vi "ChangeLanguage_old.vi"(10 "LanguageSelection":u16(ring) items=["Dansk", "English", "French"], 11 "VI Refnum":refnum<vi>) -> ()   [LabVIEW 2013, in "main.lvlib"]
uses:
  main.lvlib
  <vilib>/Utility/file.llb/Read From Spreadsheet File (string).vi
panel:
  out "Array 2":string[](array[string])
  out "appended array":string[][](array[string])
  out "Array":string[][](array[string])
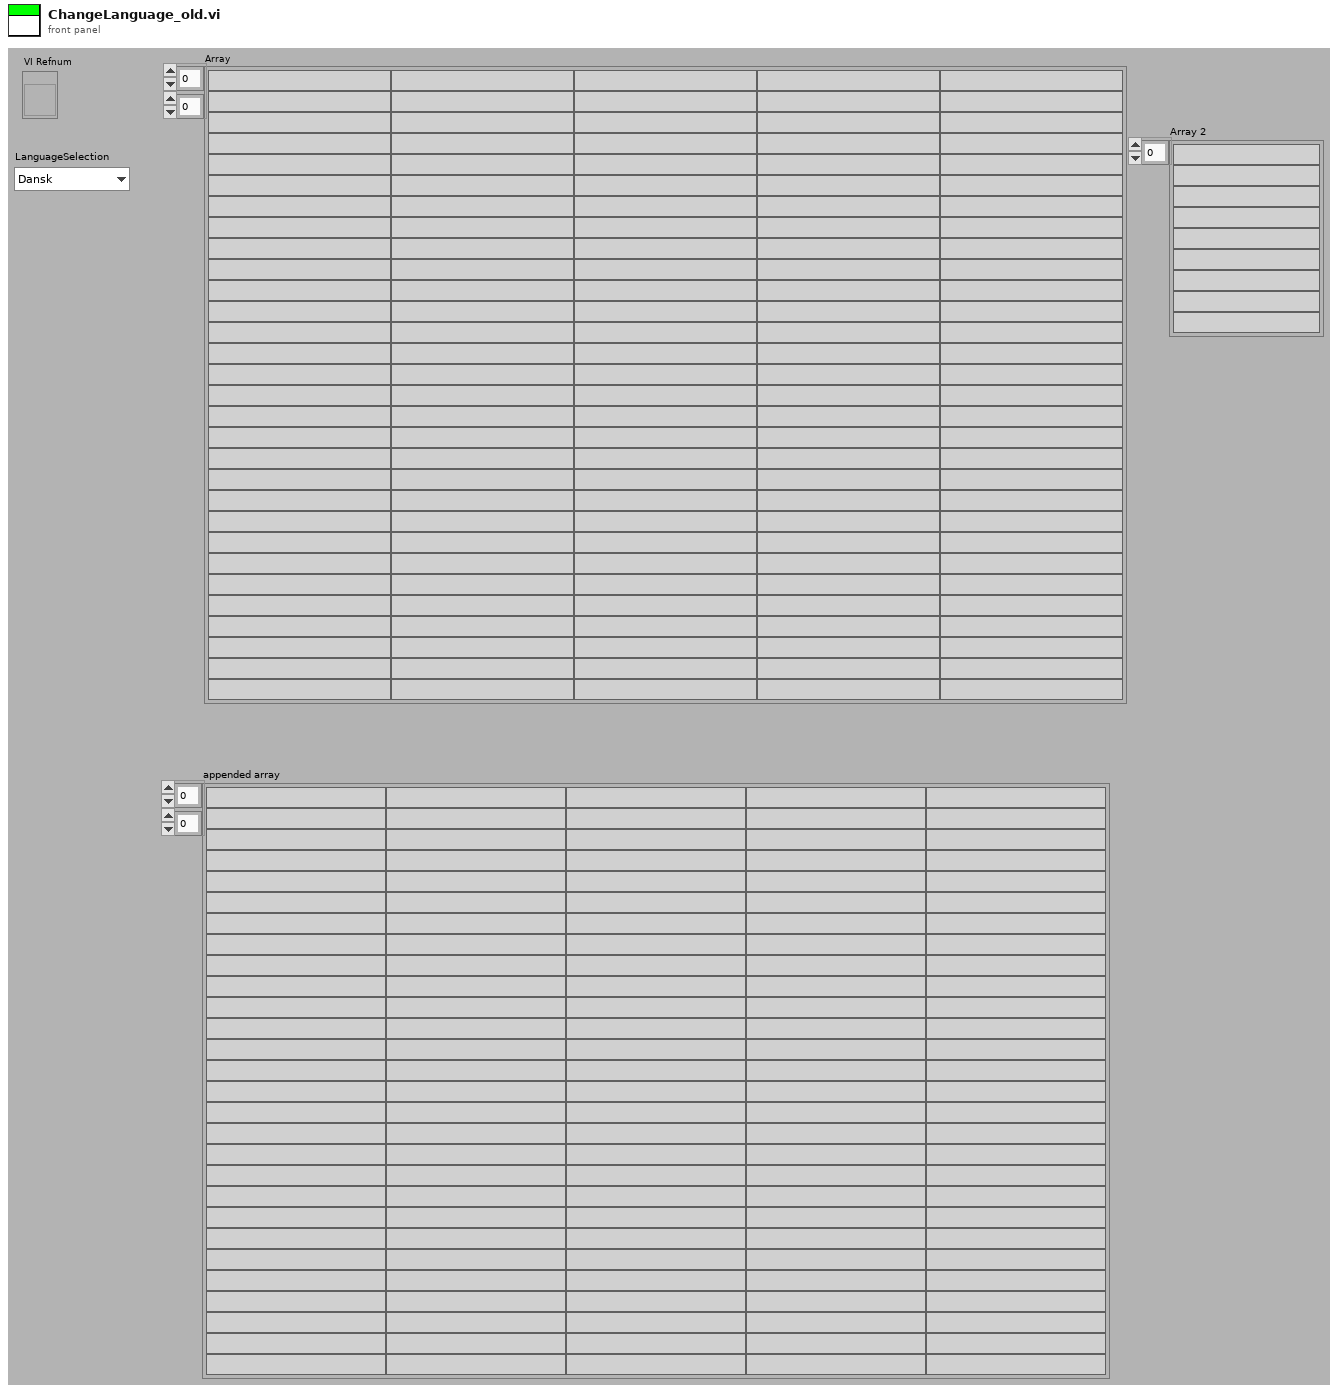
[diagram p1: front panel]
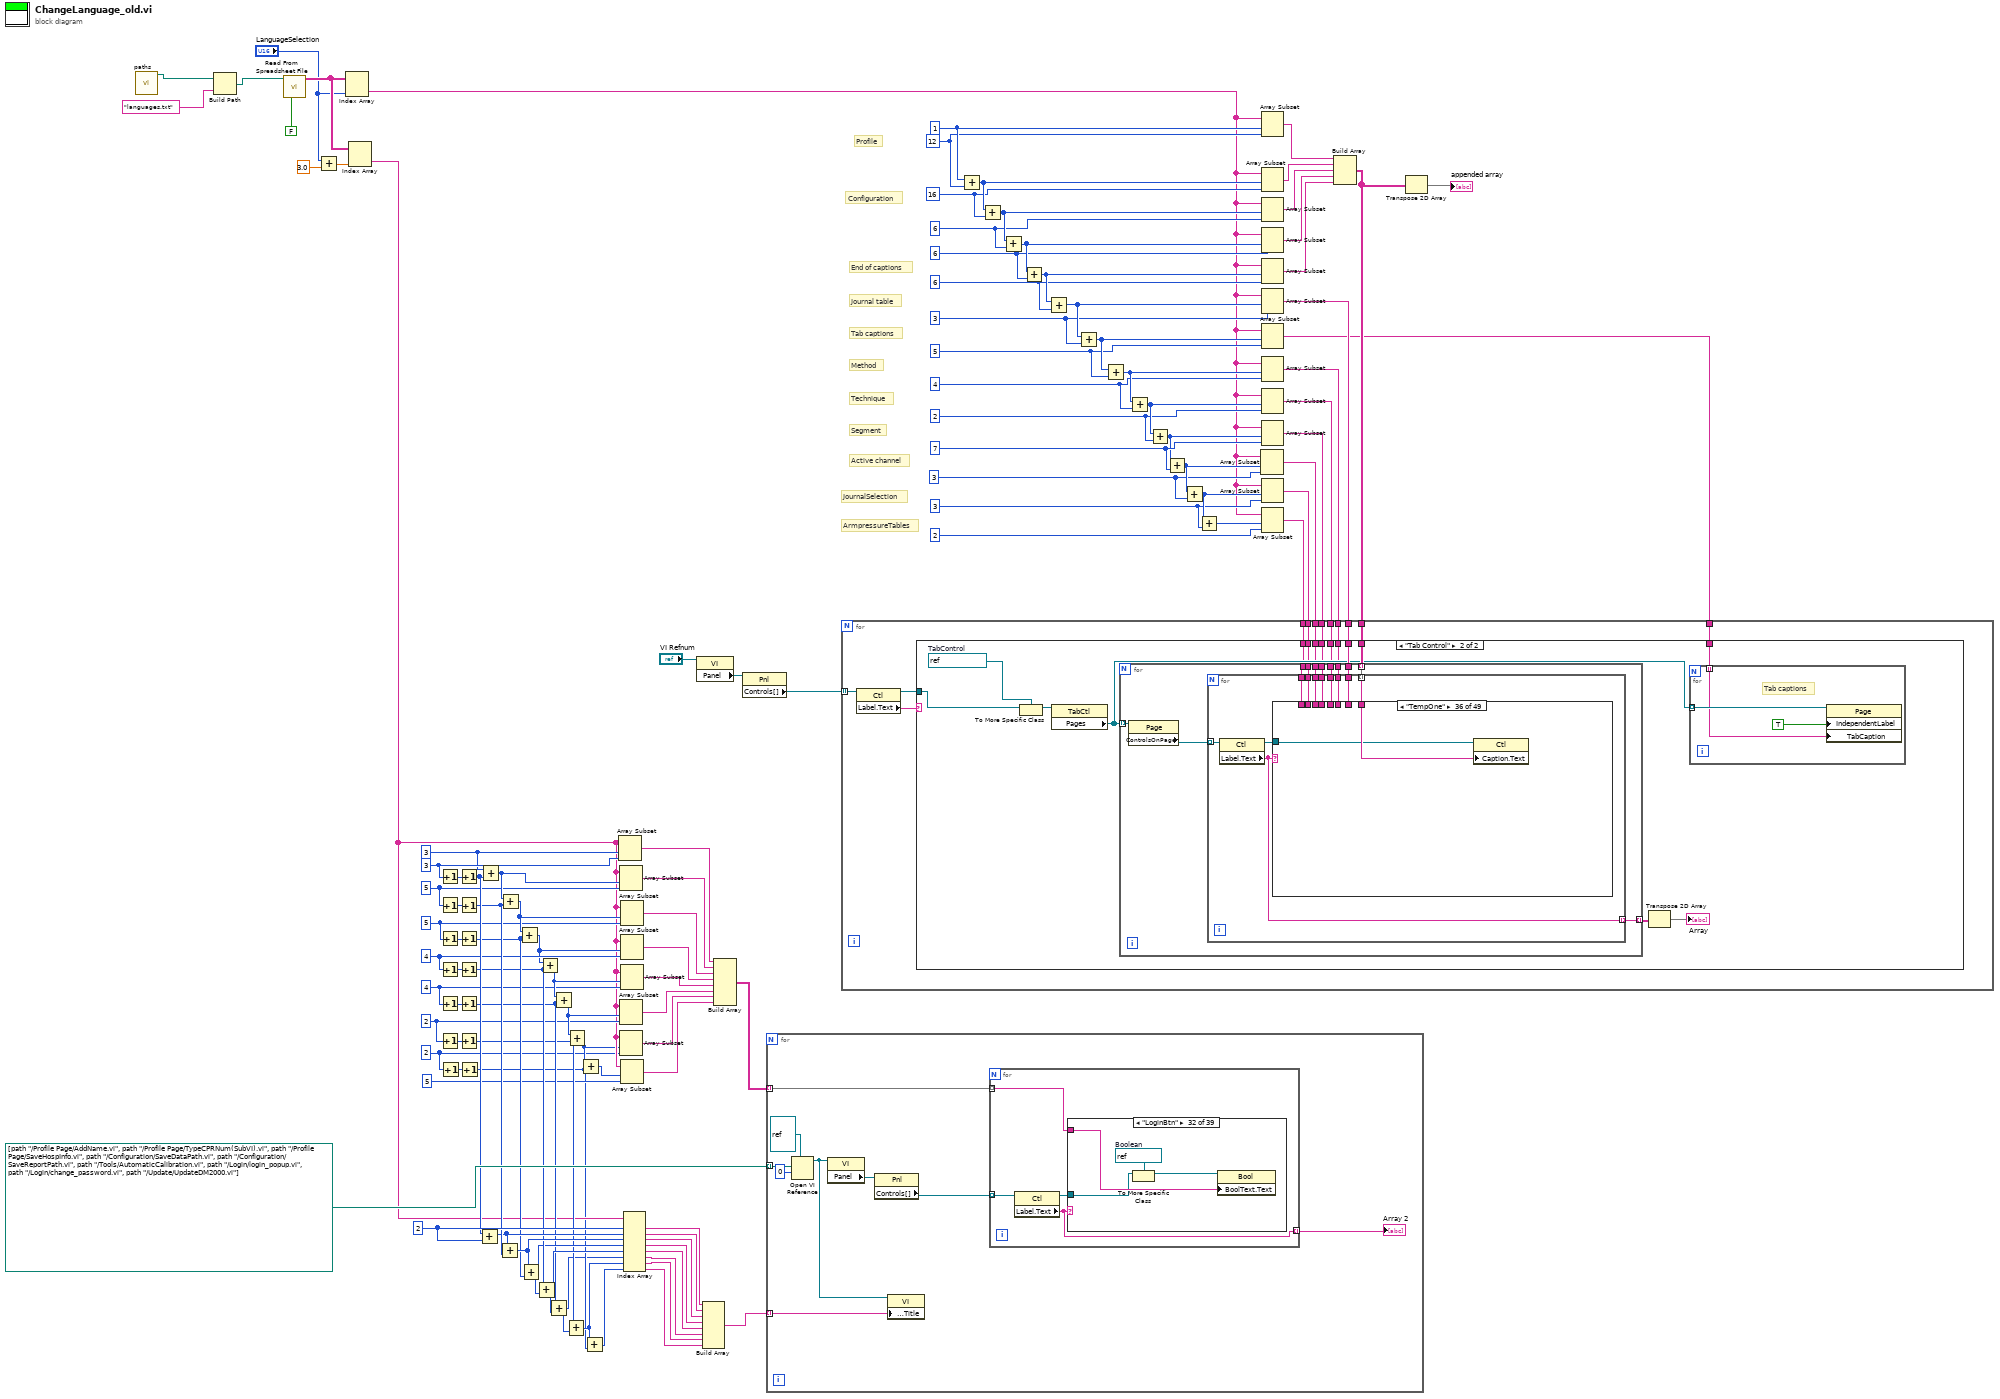
[diagram p0: block diagram]
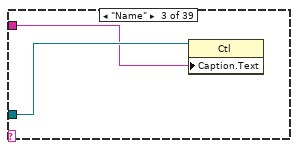
[diagram p4: hidden frame]
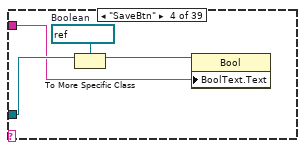
[diagram p5: hidden frame]
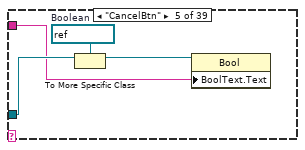
[diagram p6: hidden frame]
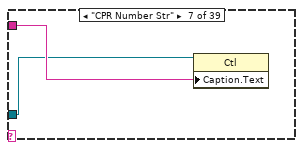
[diagram p8: hidden frame]
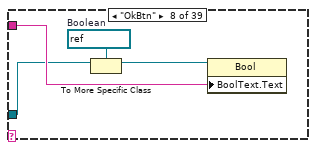
[diagram p9: hidden frame]
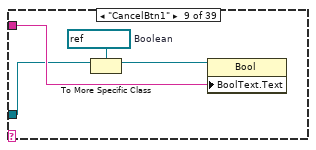
[diagram p10: hidden frame]
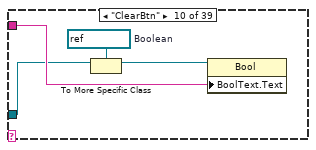
[diagram p11: hidden frame]
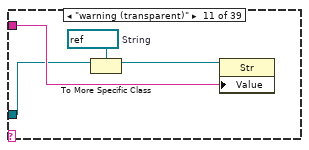
[diagram p12: hidden frame]
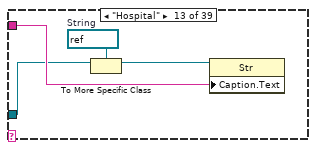
[diagram p14: hidden frame]
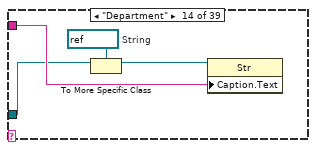
[diagram p15: hidden frame]
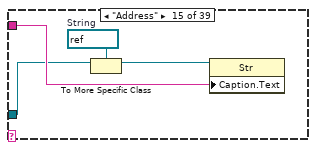
[diagram p16: hidden frame]
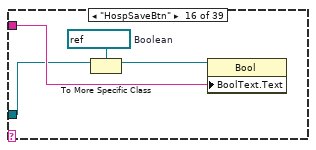
[diagram p17: hidden frame]
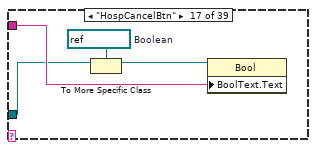
[diagram p18: hidden frame]
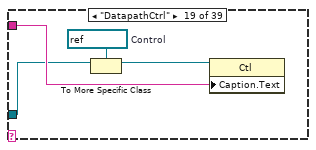
[diagram p20: hidden frame]
diagram:
  w3 = 3
  w17 = 2
  w8 = 3
  w31 = 7
  w33 = 2
  w36 = 4
  w25 = 2 ("length")
  w44 = 4 ("length")
  w53 = 4 ("length")
  w59 = 5 ("length")
  w66 = 5 ("length")
  w72 = 2 ("index")
  w71 = 3 ("length")
  w70 = 3 ("index")
  w39 = 5 ("length")
  w93 = 6 ("length")
  w95 = 16
  w87 = 3 ("length")
  w89 = 6 ("length")
  w91 = 6 ("length")
  w97 = 12 ("length")
  w98 = 1 ("index")
  # "Profile"
  # "Configuration"
  # "ArmpressureTables"
  # "JournalSelection"
  # "Tab captions"
  # "Active channel"
  # "Journal table"
  # "Segment"
  # "Technique"
  # "Method"
  # "End of captions"
  n1 = call "paths.vi"() -> ("PubAppData"=w28:path)  [unwired: 8 in, 3 out]
  n2 = Build Path(base path=w28, name or relative path="languages.txt") -> (appended path=w100:path)
  n3 = call-poly <vilib>:"Read From Spreadsheet File.vi"("transpose (no:F)"=FALSE, "file path (dialog if empty)"=w100) -> ("all rows"=w84:string[][])  [unwired: 5 in, 4 out]
  n4 = Add(x="LanguageSelection", y=3.0) -> (x+y=w83:dbl)
  n5 = Index Array(array=w84, index (col)="LanguageSelection") -> (element=w1:string[])  [unwired: 1 in]
  n6 = Index Array(array=w84, index (col)=w83) -> (element=w19:string[])  [unwired: 1 in]
  n7 = Increment(x=w71) -> (x+1=w73:i32)
  n8 = Increment(x=w66) -> (x+1=w68:i32)
  n9 = Increment(x=w59) -> (x+1=w61:i32)
  n10 = Increment(x=w53) -> (x+1=w54:i32)
  n11 = Increment(x=w44) -> (x+1=w46:i32)
  n12 = Increment(x=w25) -> (x+1=w26:i32)
  n13 = Increment(x=w17) -> (x+1=w22:i32)
  n14 = Increment(x=w73) -> (x+1=w69:i32)
  n15 = Increment(x=w68) -> (x+1=w64:i32)
  n16 = Increment(x=w61) -> (x+1=w57:i32)
  n17 = Increment(x=w54) -> (x+1=w51:i32)
  n18 = Increment(x=w46) -> (x+1=w43:i32)
  n19 = Increment(x=w26) -> (x+1=w23:i32)
  n20 = Increment(x=w22) -> (x+1=w15:i32)
  n21 = Add(x=w69, y=w72) -> (x+y=w63:i32)
  n22 = Add(x=w70, y=w69) -> (x+y=w67:i32)
  n23 = Add(x=w63, y=w64) -> (x+y=w58:i32)
  n24 = Add(x=w67, y=w64) -> (x+y=w60:i32)
  n25 = Add(x=w60, y=w57) -> (x+y=w52:i32)
  n26 = Add(x=w58, y=w57) -> (x+y=w50:i32)
  n27 = Add(x=w51, y=w50) -> (x+y=w47:i32)
  n28 = Add(x=w52, y=w51) -> (x+y=w45:i32)
  n29 = Add(x=w43, y=w47) -> (x+y=w14:i32)
  n30 = Add(x=w45, y=w43) -> (x+y=w27:i32)
  n31 = Add(x=w23, y=w14) -> (x+y=w16:i32)
  n32 = Add(x=w27, y=w23) -> (x+y=w18:i32)
  n33 = Add(x=w18, y=w15) -> (x+y=w20:i32)
  n34 = Add(x=w16, y=w15) -> (x+y=w13:i32)
  n35 = Array Subset(array=w19, index=w70, length=w71) -> (w80:string[])
  n36 = Array Subset(array=w19, index=w67, length=w66) -> (w79:string[])
  n37 = Array Subset(array=w19, index=w27, length=w25) -> (w41:string[])
  n38 = Array Subset(array=w19, index=w18, length=w17) -> (w24:string[])
  n39 = Array Subset(array=w19, index=w60, length=w59) -> (w65:string[])
  n40 = Array Subset(array=w19, index=w52, length=w53) -> (w55:string[])
  n41 = Array Subset(array=w19, index=w45, length=w44) -> (w48:string[])
  n42 = Array Subset(array=w19, index=w20, length=5) -> (w10:string[])
  n43 = Index Array(array=w19, index #1=w72, index #2=w63, index #3=w58, index #4=w50, index #5=w47, index #6=w14, index #7=w16, index #8=w13) -> (element #1=w76:string, element #2=w75:string, element #3=w62:string, element #4=w56:string, element #5=w49:string, element #6=w42:string, element #7=w12:string, element #8=w11:string)
  n44 = property class="VI"(reference="VI Refnum") -> ("Panel"=w111:refnum<vi>)  [unwired: 1 in, 2 out]
  n45 = Build Array(w76, w75, w62, w56, w49, w42, w12, w11) -> (w74:string[])
  n46 = Build Array(w80, w79, w65, w55, w48, w41, w24, w10) -> (w77:string[][])
  n47 = property class="Pnl"(reference=w111) -> ("Controls[]"=w110:refnum<vi>[])  [unwired: 1 in, 2 out]
  n48 = for {
    tunnel: path[] [path "../Profile Page/AddName.vi", path "../Profile Page/TypeCPRNum(SubVI).vi", path "../Profile Page/SaveHospInfo.vi", path "../Configuration/SaveDataPath.vi", path "../Configuration/SaveReportPath.vi", path "../Tools/AutomaticCalibration.vi", path "../Login/login_popup.vi", path "../Login/change_password.vi", path "../Update/UpdateDM2000.vi"] -> [w120] mode=indexing
    tunnel: w77 -> [w113] mode=indexing
    tunnel: w74 -> [w112] mode=indexing
    n49 = Open VI Reference(type specifier VI Refnum (for type only)=refnum<vi> refnum, vi path=w120, options=0) -> (vi reference=w114:refnum<vi>)  [unwired: 3 in, 1 out]
    n50 = property class="VI"(reference=w114) -> ("Panel"=w117:refnum<vi>)  [unwired: 1 in, 2 out]
    n51 = property class="Pnl"(reference=w117) -> ("Controls[]"=w119:refnum<vi>[])  [unwired: 1 in, 2 out]
    n52 = property class="VI"(reference=w114, "Front Panel.Title"=w112) -> ()  [unwired: 1 in, 2 out]
    n53 = for {
      tunnel: w119 -> [w124] mode=indexing
      tunnel: [w122] -> w118 mode=indexing
      tunnel: w113 -> [w121] mode=indexing
      n54 = property class="Ctl"(reference=w124) -> (reference out=w123:refnum<vi>, "Label.Text"=w122:string)  [unwired: 1 in, 1 out]
      n55 = case shown="\"LoginBtn\"" w122 {
        tunnel: w123 -> [_ _ w126 w129 w133 _ w135 w137 w141 w145 w149 _ w153 w157 w161 w165 w169 _ w173 w177 w181 w185 _ w189 w193 w197 w201 _ w205 w209 _ w213 w217 _ w221 w225 w229 w233 w237]
        tunnel: w121 -> [_ _ w125 w127 w131 _ w136 w138 w142 w146 w150 _ w154 w158 w162 w166 w170 _ w174 w178 w182 w186 _ w190 w194 w198 w202 _ w206 w210 _ w214 w218 _ w222 w226 w230 w234 w238]
        frame Default {
        }
        frame "/**AddName.vi" {
        }
        frame "Name" {
          n56 = property class="Ctl"(reference=w126, "Caption.Text"=w125) -> ()  [unwired: 1 in, 2 out]
        }
        frame "SaveBtn" {
          w130 = refnum<vi> refnum  # Boolean
          n57 = To More Specific Class(target class=w130, reference=w129) -> (specific class reference=w128:refnum<vi>)  [unwired: 1 in, 1 out]
          n58 = property class="Bool"(reference=w128, "BoolText.Text"=w127) -> ()  [unwired: 1 in, 2 out]
        }
        frame "CancelBtn" {
          w134 = refnum<vi> refnum  # Boolean
          n59 = To More Specific Class(target class=w134, reference=w133) -> (specific class reference=w132:refnum<vi>)  [unwired: 1 in, 1 out]
          n60 = property class="Bool"(reference=w132, "BoolText.Text"=w131) -> ()  [unwired: 1 in, 2 out]
        }
        frame "/**TypeCPRNum" {
        }
        frame "CPR Number Str" {
          n61 = property class="Ctl"(reference=w135, "Caption.Text"=w136) -> ()  [unwired: 1 in, 2 out]
        }
        frame "OkBtn" {
          w140 = refnum<vi> refnum  # Boolean
          n62 = To More Specific Class(target class=w140, reference=w137) -> (specific class reference=w139:refnum<vi>)  [unwired: 1 in, 1 out]
          n63 = property class="Bool"(reference=w139, "BoolText.Text"=w138) -> ()  [unwired: 1 in, 2 out]
        }
        frame "CancelBtn1" {
          w144 = refnum<vi> refnum  # Boolean
          n64 = To More Specific Class(target class=w144, reference=w141) -> (specific class reference=w143:refnum<vi>)  [unwired: 1 in, 1 out]
          n65 = property class="Bool"(reference=w143, "BoolText.Text"=w142) -> ()  [unwired: 1 in, 2 out]
        }
        frame "ClearBtn" {
          w148 = refnum<vi> refnum  # Boolean
          n66 = To More Specific Class(target class=w148, reference=w145) -> (specific class reference=w147:refnum<vi>)  [unwired: 1 in, 1 out]
          n67 = property class="Bool"(reference=w147, "BoolText.Text"=w146) -> ()  [unwired: 1 in, 2 out]
        }
        frame "warning (transparent)" {
          w152 = refnum<vi> refnum  # String
          n68 = To More Specific Class(target class=w152, reference=w149) -> (specific class reference=w151:refnum<vi>)  [unwired: 1 in, 1 out]
          n69 = property class="Str"(reference=w151, "Value"=w150) -> ()  [unwired: 1 in, 2 out]
        }
        frame "/***HospInfo" {
        }
        frame "Hospital" {
          w156 = refnum<vi> refnum  # String
          n70 = To More Specific Class(target class=w156, reference=w153) -> (specific class reference=w155:refnum<vi>)  [unwired: 1 in, 1 out]
          n71 = property class="Str"(reference=w155, "Caption.Text"=w154) -> ()  [unwired: 1 in, 2 out]
        }
        frame "Department" {
          w160 = refnum<vi> refnum  # String
          n72 = To More Specific Class(target class=w160, reference=w157) -> (specific class reference=w159:refnum<vi>)  [unwired: 1 in, 1 out]
          n73 = property class="Str"(reference=w159, "Caption.Text"=w158) -> ()  [unwired: 1 in, 2 out]
        }
        frame "Address" {
          w164 = refnum<vi> refnum  # String
          n74 = To More Specific Class(target class=w164, reference=w161) -> (specific class reference=w163:refnum<vi>)  [unwired: 1 in, 1 out]
          n75 = property class="Str"(reference=w163, "Caption.Text"=w162) -> ()  [unwired: 1 in, 2 out]
        }
        frame "HospSaveBtn" {
          w168 = refnum<vi> refnum  # Boolean
          n76 = To More Specific Class(target class=w168, reference=w165) -> (specific class reference=w167:refnum<vi>)  [unwired: 1 in, 1 out]
          n77 = property class="Bool"(reference=w167, "BoolText.Text"=w166) -> ()  [unwired: 1 in, 2 out]
        }
        frame "HospCancelBtn" {
          w172 = refnum<vi> refnum  # Boolean
          n78 = To More Specific Class(target class=w172, reference=w169) -> (specific class reference=w171:refnum<vi>)  [unwired: 1 in, 1 out]
          n79 = property class="Bool"(reference=w171, "BoolText.Text"=w170) -> ()  [unwired: 1 in, 2 out]
        }
        frame "/***SaveDataPath" {
        }
        frame "DatapathCtrl" {
          w176 = refnum<vi> refnum  # Control
          n80 = To More Specific Class(target class=w176, reference=w173) -> (specific class reference=w175:refnum<vi>)  [unwired: 1 in, 1 out]
          n81 = property class="Ctl"(reference=w175, "Caption.Text"=w174) -> ()  [unwired: 1 in, 2 out]
        }
        frame "DatapathSaveBtn" {
          w180 = refnum<vi> refnum  # Boolean
          n82 = To More Specific Class(target class=w180, reference=w177) -> (specific class reference=w179:refnum<vi>)  [unwired: 1 in, 1 out]
          n83 = property class="Bool"(reference=w179, "BoolText.Text"=w178) -> ()  [unwired: 1 in, 2 out]
        }
        frame "DatapathCancelBtn" {
          w184 = refnum<vi> refnum  # Boolean
          n84 = To More Specific Class(target class=w184, reference=w181) -> (specific class reference=w183:refnum<vi>)  [unwired: 1 in, 1 out]
          n85 = property class="Bool"(reference=w183, "BoolText.Text"=w182) -> ()  [unwired: 1 in, 2 out]
        }
        frame "String (transparent)" {
          w188 = refnum<vi> refnum  # String
          n86 = To More Specific Class(target class=w188, reference=w185) -> (specific class reference=w187:refnum<vi>)  [unwired: 1 in, 1 out]
          n87 = property class="Str"(reference=w187, "Caption.Text"=w186) -> ()  [unwired: 1 in, 2 out]
        }
        frame "/***SaveReportPath" {
        }
        frame "ReportPathCtrl" {
          w192 = refnum<vi> refnum  # Control
          n88 = To More Specific Class(target class=w192, reference=w189) -> (specific class reference=w191:refnum<vi>)  [unwired: 1 in, 1 out]
          n89 = property class="Ctl"(reference=w191, "Caption.Text"=w190) -> ()  [unwired: 1 in, 2 out]
        }
        frame "ReportSaveBtn" {
          w196 = refnum<vi> refnum  # Boolean
          n90 = To More Specific Class(target class=w196, reference=w193) -> (specific class reference=w195:refnum<vi>)  [unwired: 1 in, 1 out]
          n91 = property class="Bool"(reference=w195, "BoolText.Text"=w194) -> ()  [unwired: 1 in, 2 out]
        }
        frame "ReportCancelBtn" {
          w200 = refnum<vi> refnum  # Boolean
          n92 = To More Specific Class(target class=w200, reference=w197) -> (specific class reference=w199:refnum<vi>)  [unwired: 1 in, 1 out]
          n93 = property class="Bool"(reference=w199, "BoolText.Text"=w198) -> ()  [unwired: 1 in, 2 out]
        }
        frame "ReportString (transparent)" {
          w204 = refnum<vi> refnum  # String
          n94 = To More Specific Class(target class=w204, reference=w201) -> (specific class reference=w203:refnum<vi>)  [unwired: 1 in, 1 out]
          n95 = property class="Str"(reference=w203, "Caption.Text"=w202) -> ()  [unwired: 1 in, 2 out]
        }
        frame "/***AutomaticCalibration" {
        }
        frame "CalibrationStopBtn" {
          w208 = refnum<vi> refnum  # Boolean
          n96 = To More Specific Class(target class=w208, reference=w205) -> (specific class reference=w207:refnum<vi>)  [unwired: 1 in, 1 out]
          n97 = property class="Bool"(reference=w207, "BoolText.Text"=w206) -> ()  [unwired: 1 in, 2 out]
        }
        frame "CalibrationCancelBtn" {
          w212 = refnum<vi> refnum  # Boolean
          n98 = To More Specific Class(target class=w212, reference=w209) -> (specific class reference=w211:refnum<vi>)  [unwired: 1 in, 1 out]
          n99 = property class="Bool"(reference=w211, "BoolText.Text"=w210) -> ()  [unwired: 1 in, 2 out]
        }
        frame "/**Login**/" {
        }
        frame "LoginBtn" {
          w216 = refnum<vi> refnum  # Boolean
          n100 = To More Specific Class(target class=w216, reference=w213) -> (specific class reference=w215:refnum<vi>)  [unwired: 1 in, 1 out]
          n101 = property class="Bool"(reference=w215, "BoolText.Text"=w214) -> ()  [unwired: 1 in, 2 out]
        }
        frame "LoginCancelBtn" {
          w220 = refnum<vi> refnum  # Boolean
          n102 = To More Specific Class(target class=w220, reference=w217) -> (specific class reference=w219:refnum<vi>)  [unwired: 1 in, 1 out]
          n103 = property class="Bool"(reference=w219, "BoolText.Text"=w218) -> ()  [unwired: 1 in, 2 out]
        }
        frame "/**ChangePassword**/" {
        }
        frame "PresentPassword" {
          w224 = refnum<vi> refnum  # String
          n104 = To More Specific Class(target class=w224, reference=w221) -> (specific class reference=w223:refnum<vi>)  [unwired: 1 in, 1 out]
          n105 = property class="Str"(reference=w223, "Caption.Text"=w222) -> ()  [unwired: 1 in, 2 out]
        }
        frame "NewPassword" {
          w228 = refnum<vi> refnum  # String
          n106 = To More Specific Class(target class=w228, reference=w225) -> (specific class reference=w227:refnum<vi>)  [unwired: 1 in, 1 out]
          n107 = property class="Str"(reference=w227, "Caption.Text"=w226) -> ()  [unwired: 1 in, 2 out]
        }
        frame "RetypePassword" {
          w232 = refnum<vi> refnum  # String
          n108 = To More Specific Class(target class=w232, reference=w229) -> (specific class reference=w231:refnum<vi>)  [unwired: 1 in, 1 out]
          n109 = property class="Str"(reference=w231, "Caption.Text"=w230) -> ()  [unwired: 1 in, 2 out]
        }
        frame "Submit" {
          w236 = refnum<vi> refnum  # Boolean
          n110 = To More Specific Class(target class=w236, reference=w233) -> (specific class reference=w235:refnum<vi>)  [unwired: 1 in, 1 out]
          n111 = property class="Bool"(reference=w235, "BoolText.Text"=w234) -> ()  [unwired: 1 in, 2 out]
        }
        frame "Cancel" {
          w240 = refnum<vi> refnum  # Boolean
          n112 = To More Specific Class(target class=w240, reference=w237) -> (specific class reference=w239:refnum<vi>)  [unwired: 1 in, 1 out]
          n113 = property class="Bool"(reference=w239, "BoolText.Text"=w238) -> ()  [unwired: 1 in, 2 out]
        }
      }
    }
    "Array 2" <- w118
  }
  n114 = Add(x=w98, y=w97) -> (x+y=w96:i32)
  n115 = Add(x=w96, y=w95) -> (x+y=w94:i32)
  n116 = Add(x=w94, y=w93) -> (x+y=w92:i32)
  n117 = Add(x=w92, y=w91) -> (x+y=w90:i32)
  n118 = Add(x=w90, y=w89) -> (x+y=w88:i32)
  n119 = Add(x=w88, y=w87) -> (x+y=w40:i32)
  n120 = Add(x=w40, y=w39) -> (x+y=w37:i32)
  n121 = Add(x=w37, y=w36) -> (x+y=w34:i32)
  n122 = Add(x=w34, y=w33) -> (x+y=w30:i32)
  n123 = Add(x=w30, y=w31) -> (x+y=w9:i32)
  n124 = Add(x=w9, y=w8) -> (x+y=w4:i32)
  n125 = Add(x=w4, y=w3) -> (x+y=w6:i32)
  n126 = Array Subset(array=w1, index=w9, length=w8) -> (w29:string[])
  n127 = Array Subset(array=w1, index=w98, length=w97) -> (w108:string[])
  n128 = Array Subset(array=w1, index=w96, length=w95) -> (w107:string[])
  n129 = Array Subset(array=w1, index=w94, length=w93) -> (w106:string[])
  n130 = Array Subset(array=w1, index=w92, length=w91) -> (w105:string[])
  n131 = Array Subset(array=w1, index=w90, length=w89) -> (w104:string[])
  n132 = Array Subset(array=w1, index=w88, length=w87) -> (w101:string[])
  n133 = Array Subset(array=w1, index=w40, length=w39) -> (w86:string[])
  n134 = Array Subset(array=w1, index=w37, length=w36) -> (w38:string[])
  n135 = Array Subset(array=w1, index=w34, length=w33) -> (w35:string[])
  n136 = Array Subset(array=w1, index=w30, length=w31) -> (w32:string[])
  n137 = Array Subset(array=w1, index=w4, length=w3) -> (w7:string[])
  n138 = Array Subset(array=w1, index=w6, length=2) -> (w2:string[])
  n139 = Build Array(w108, w107, w106, w105, w104) -> (w102:string[][])
  n140 = for {
    tunnel: w110 -> [w252] mode=indexing
    tunnel: w102 -> [w249]
    tunnel: w101 -> [w248]
    tunnel: w86 -> [w247]
    tunnel: w38 -> [w246]
    tunnel: w35 -> [w245]
    tunnel: w32 -> [w244]
    tunnel: w29 -> [w243]
    tunnel: w7 -> [w242]
    tunnel: w2 -> [w241]
    n141 = property class="Ctl"(reference=w252) -> (reference out=w251:refnum<vi>, "Label.Text"=w250:string)  [unwired: 1 in, 1 out]
    n142 = case shown="\"Tab Control\"" w250 {
      tunnel: w251 -> [_ w267]
      tunnel: w249 -> [_ w262]
      tunnel: w248 -> [_ w261]
      tunnel: w247 -> [_ w259]
      tunnel: w246 -> [_ w258]
      tunnel: w245 -> [_ w257]
      tunnel: w244 -> [_ w256]
      tunnel: w243 -> [_ w255]
      tunnel: w242 -> [_ w254]
      tunnel: w241 -> [_ w253]
      frame "False", Default {
      }
      frame "Tab Control" {
        w266 = refnum<vi> refnum  # TabControl
        n143 = To More Specific Class(target class=w266, reference=w267) -> (specific class reference=w265:refnum<vi>)  [unwired: 1 in, 1 out]
        n144 = property class="TabCtl"(reference=w265) -> ("Pages"=w260:refnum<vi>[])  [unwired: 1 in, 2 out]
        n145 = for {
          tunnel: w260 -> [w277] mode=indexing
          tunnel: [w280] -> w264 mode=indexing
          tunnel: w262 -> [w279] mode=indexing
          tunnel: w261 -> [w278]
          tunnel: w258 -> [w276]
          tunnel: w257 -> [w275]
          tunnel: w256 -> [w274]
          tunnel: w255 -> [w273]
          tunnel: w254 -> [w272]
          tunnel: w253 -> [w271]
          n146 = property class="Page"(reference=w277) -> ("ControlsOnPage"=w281:refnum<vi>[])  [unwired: 1 in, 2 out]
          n147 = for {
            tunnel: w281 -> [w292] mode=indexing
            tunnel: [w291] -> w280 mode=indexing
            tunnel: w279 -> [w289] mode=indexing
            tunnel: w278 -> [w288]
            tunnel: w276 -> [w287]
            tunnel: w275 -> [w286]
            tunnel: w274 -> [w285]
            tunnel: w273 -> [w284]
            tunnel: w272 -> [w283]
            tunnel: w271 -> [w282]
            n148 = property class="Ctl"(reference=w292) -> (reference out=w290:refnum<vi>, "Label.Text"=w291:string)  [unwired: 1 in, 1 out]
            n149 = case shown="\"TempOne\"" w291 {
              tunnel: w290 -> [_ w295 w298 w302 w303 w309 w312 w316 w318 w322 w324 w326 w328 w331 w336 w341 w345 w347 w351 w356 w359 w361 w363 w365 w369 w373 w377 w380 w382 w384 w386 w388 w390 w392 w394 w396 w398 w400 w402 w404 w408 w413 w415 w419 w424 w427 w431 w435 w439]
              tunnel: w289 -> [_ w296 w300 w301 w306 w308 w311 w315 w320 w321 w323 w325 w327 w330 w335 w340 w344 w346 w349 w354 w358 w360 w362 w364 w368 w372 w376 w381 w383 w385 w387 w389 w391 w393 w395 w397 w399 w401 w403 w405 w410 w412 w416 w420 w425 w426 w430 _ w440]
              tunnel: w288 -> [_ _ _ _ _ _ _ _ _ _ _ _ _ _ _ _ _ _ _ _ _ _ _ _ _ _ _ _ _ _ _ _ _ _ _ _ _ _ _ _ _ _ _ _ _ _ _ w434 _]
              tunnel: w287 -> [_ _ _ _ _ _ _ _ _ _ _ _ _ w329 _ _ _ _ _ _ _ _ _ _ _ _ _ _ _ _ _ _ _ _ _ _ _ _ _ _ _ _ _ _ _ _ _ _ _]
              tunnel: w286 -> [_ _ _ _ _ _ _ _ _ _ _ _ _ _ w334 _ _ _ _ _ _ _ _ _ _ _ _ _ _ _ _ _ _ _ _ _ _ _ _ _ _ _ _ _ _ _ _ _ _]
              tunnel: w285 -> [_ _ _ _ _ _ _ _ _ _ _ _ _ _ _ w339 _ _ _ _ _ _ _ _ _ _ _ _ _ _ _ _ _ _ _ _ _ _ _ _ _ _ _ _ _ _ _ _ _]
              tunnel: w284 -> [_ _ _ _ _ _ _ _ _ _ _ _ _ _ _ _ _ _ _ _ _ _ _ _ _ _ _ _ _ _ _ _ _ _ _ _ _ _ _ _ w406 _ _ _ _ _ _ _ _]
              tunnel: w283 -> [_ _ _ _ _ _ _ _ _ _ _ _ _ _ _ _ _ _ _ _ _ _ _ _ _ _ _ _ _ _ _ _ _ _ _ _ _ _ _ _ _ _ _ _ w421 _ _ _ _]
              tunnel: w282 -> [_ _ _ _ _ _ _ _ _ _ _ _ _ _ _ _ _ _ w348 w353 _ _ _ _ _ _ _ _ _ _ _ _ _ _ _ _ _ _ _ _ _ _ _ _ _ _ _ _ _]
              frame Default {
              }
              frame "ListboxCpr" {
                w294 = refnum<vi> refnum  # ListBox
                n150 = To More Specific Class(target class=w294, reference=w295) -> (specific class reference=w293:refnum<vi>)  [unwired: 1 in, 1 out]
                n151 = property class="LstBox"(reference=w293, "ColHdr"=w296) -> ()  [unwired: 1 in, 2 out]
              }
              frame "SelectCprBtn" {
                w299 = refnum<vi> refnum  # Boolean
                n152 = To More Specific Class(target class=w299, reference=w298) -> (specific class reference=w297:refnum<vi>)  [unwired: 1 in, 1 out]
                n153 = property class="Bool"(reference=w297, "BoolText.Text"=w300) -> ()  [unwired: 1 in, 2 out]
              }
              frame "Name" {
                n154 = property class="Ctl"(reference=w302, "Caption.Text"=w301) -> ()  [unwired: 1 in, 2 out]
              }
              frame "AddCprBtn" {
                w305 = refnum<vi> refnum  # Boolean
                n155 = To More Specific Class(target class=w305, reference=w303) -> (specific class reference=w304:refnum<vi>)  [unwired: 1 in, 1 out]
                n156 = property class="Bool"(reference=w304, "BoolText.Text"=w306) -> ()  [unwired: 1 in, 2 out]
              }
              frame "ListboxOperator" {
                w310 = refnum<vi> refnum  # ListBox
                n157 = To More Specific Class(target class=w310, reference=w309) -> (specific class reference=w307:refnum<vi>)  [unwired: 1 in, 1 out]
                n158 = property class="LstBox"(reference=w307, "ColHdr"=w308) -> ()  [unwired: 1 in, 2 out]
              }
              frame "ListboxDoctor" {
                w314 = refnum<vi> refnum  # ListBox
                n159 = To More Specific Class(target class=w314, reference=w312) -> (specific class reference=w313:refnum<vi>)  [unwired: 1 in, 1 out]
                n160 = property class="LstBox"(reference=w313, "ColHdr"=w311) -> ()  [unwired: 1 in, 2 out]
              }
              frame "HospitalName" {
                n161 = property class="Ctl"(reference=w316, "Caption.Text"=w315) -> ()  [unwired: 1 in, 2 out]
              }
              frame "EditHospInfo" {
                w319 = refnum<vi> refnum  # Boolean
                n162 = To More Specific Class(target class=w319, reference=w318) -> (specific class reference=w317:refnum<vi>)  [unwired: 1 in, 1 out]
                n163 = property class="Bool"(reference=w317, "BoolText.Text"=w320) -> ()  [unwired: 1 in, 2 out]
              }
              frame "HospitalAddress" {
                n164 = property class="Ctl"(reference=w322, "Caption.Text"=w321) -> ()  [unwired: 1 in, 2 out]
              }
              frame "CommentString" {
                n165 = property class="Ctl"(reference=w324, "Caption.Text"=w323) -> ()  [unwired: 1 in, 2 out]
              }
              frame "HospitalDepartment" {
                n166 = property class="Ctl"(reference=w326, "Caption.Text"=w325) -> ()  [unwired: 1 in, 2 out]
              }
              frame "SearchCprField" {
                n167 = property class="Ctl"(reference=w328, "Caption.Text"=w327) -> ()  [unwired: 1 in, 2 out]
              }
              frame "ListboxMeasurementMeth" {
                w333 = refnum<vi> refnum  # ListBox
                n168 = To More Specific Class(target class=w333, reference=w331) -> (specific class reference=w332:refnum<vi>)  [unwired: 1 in, 1 out]
                n169 = property class="LstBox"(reference=w332, "Caption.Text"=w330, "Item Names"=w329) -> ()  [unwired: 1 in, 2 out]
              }
              frame "ListboxMeasurementTechnique" {
                w338 = refnum<vi> refnum  # ListBox
                n170 = To More Specific Class(target class=w338, reference=w336) -> (specific class reference=w337:refnum<vi>)  [unwired: 1 in, 1 out]
                n171 = property class="LstBox"(reference=w337, "Caption.Text"=w335, "Item Names"=w334) -> ()  [unwired: 1 in, 2 out]
              }
              frame "ListboxMeasurementArea" {
                w343 = refnum<vi> refnum  # ListBox
                n172 = To More Specific Class(target class=w343, reference=w341) -> (specific class reference=w342:refnum<vi>)  [unwired: 1 in, 1 out]
                n173 = property class="LstBox"(reference=w342, "Caption.Text"=w340, "Item Names"=w339) -> ()  [unwired: 1 in, 2 out]
              }
              frame "ListboxRightSegmentNr" {
                n174 = property class="Ctl"(reference=w345, "Caption.Text"=w344) -> ()  [unwired: 1 in, 2 out]
              }
              frame "ListboxLeftSegmentNr" {
                n175 = property class="Ctl"(reference=w347, "Caption.Text"=w346) -> ()  [unwired: 1 in, 2 out]
              }
              frame "RightArmPressureTable" {
                w350 = refnum<vi> refnum  # Table
                n176 = To More Specific Class(target class=w350, reference=w351) -> (specific class reference=w352:refnum<vi>)  [unwired: 1 in, 1 out]
                n177 = property class="Tbl"(reference=w352, "Caption.Text"=w349, "Column Headers[]"=w348) -> ()  [unwired: 1 in, 2 out]
              }
              frame "LeftArmPressureTable" {
                w355 = refnum<vi> refnum  # Table
                n178 = To More Specific Class(target class=w355, reference=w356) -> (specific class reference=w357:refnum<vi>)  [unwired: 1 in, 1 out]
                n179 = property class="Tbl"(reference=w357, "Caption.Text"=w354, "Column Headers[]"=w353) -> ()  [unwired: 1 in, 2 out]
              }
              frame "Puls" {
                n180 = property class="Ctl"(reference=w359, "Caption.Text"=w358) -> ()  [unwired: 1 in, 2 out]
              }
              frame "HeightAdjustmentInt" {
                n181 = property class="Ctl"(reference=w361, "Caption.Text"=w360) -> ()  [unwired: 1 in, 2 out]
              }
              frame "Segment Number" {
                n182 = property class="Ctl"(reference=w363, "Caption.Text"=w362) -> ()  [unwired: 1 in, 2 out]
              }
              frame "SaveArmPressureBtn" {
                w367 = refnum<vi> refnum  # Boolean
                n183 = To More Specific Class(target class=w367, reference=w365) -> (specific class reference=w366:refnum<vi>)  [unwired: 1 in, 1 out]
                n184 = property class="Bool"(reference=w366, "BoolText.Text"=w364) -> ()  [unwired: 1 in, 2 out]
              }
              frame "EditDataPath" {
                w371 = refnum<vi> refnum  # Boolean
                n185 = To More Specific Class(target class=w371, reference=w369) -> (specific class reference=w370:refnum<vi>)  [unwired: 1 in, 1 out]
                n186 = property class="Bool"(reference=w370, "BoolText.Text"=w368) -> ()  [unwired: 1 in, 2 out]
              }
              frame "ReportPathBtn" {
                w375 = refnum<vi> refnum  # Boolean
                n187 = To More Specific Class(target class=w375, reference=w373) -> (specific class reference=w374:refnum<vi>)  [unwired: 1 in, 1 out]
                n188 = property class="Bool"(reference=w374, "BoolText.Text"=w372) -> ()  [unwired: 1 in, 2 out]
              }
              frame "ChangeLanguage" {
                w379 = refnum<vi> refnum  # Ring
                n189 = To More Specific Class(target class=w379, reference=w377) -> (specific class reference=w378:refnum<vi>)  [unwired: 1 in, 1 out]
                n190 = property class="Ring"(reference=w378, "Caption.Text"=w376) -> ()  [unwired: 1 in, 2 out]
              }
              frame "Arm1" {
                n191 = property class="Ctl"(reference=w380, "Value"=w381) -> ()  [unwired: 1 in, 2 out]
              }
              frame "Arm2" {
                n192 = property class="Ctl"(reference=w382, "Value"=w383) -> ()  [unwired: 1 in, 2 out]
              }
              frame "Right1" {
                n193 = property class="Ctl"(reference=w384, "Value"=w385) -> ()  [unwired: 1 in, 2 out]
              }
              frame "Left1" {
                n194 = property class="Ctl"(reference=w386, "Value"=w387) -> ()  [unwired: 1 in, 2 out]
              }
              frame "Right2" {
                n195 = property class="Ctl"(reference=w388, "Value"=w389) -> ()  [unwired: 1 in, 2 out]
              }
              frame "Left2" {
                n196 = property class="Ctl"(reference=w390, "Value"=w391) -> ()  [unwired: 1 in, 2 out]
              }
              frame "SettingsString" {
                n197 = property class="Ctl"(reference=w392, "Value"=w393) -> ()  [unwired: 1 in, 2 out]
              }
              frame "AdditionalInfoString" {
                n198 = property class="Ctl"(reference=w394, "Caption.Text"=w395) -> ()  [unwired: 1 in, 2 out]
              }
              frame "TempOne" {
                n199 = property class="Ctl"(reference=w396, "Caption.Text"=w397) -> ()  [unwired: 1 in, 2 out]
              }
              frame "AutoCompleteArmPresBool" {
                n200 = property class="Ctl"(reference=w398, "Caption.Text"=w399) -> ()  [unwired: 1 in, 2 out]
              }
              frame "Calibration" {
                n201 = property class="Ctl"(reference=w400, "Caption.Text"=w401) -> ()  [unwired: 1 in, 2 out]
              }
              frame "AcqTestBtn" {
                n202 = property class="Ctl"(reference=w402, "Caption.Text"=w403) -> ()  [unwired: 1 in, 2 out]
              }
              frame "AcqFilt" {
                n203 = property class="Ctl"(reference=w404, "Caption.Text"=w405) -> ()  [unwired: 1 in, 2 out]
              }
              frame "RingActGraph" {
                w407 = refnum<vi> refnum  # Ring
                n204 = To More Specific Class(target class=w407, reference=w408) -> (specific class reference=w409:refnum<vi>)  [unwired: 1 in, 1 out]
                n205 = property class="Ring"(reference=w409, "Caption.Text"=w410, "Strings []"=w406) -> ()  [unwired: 1 in, 2 out]
              }
              frame "GraphSelection" {
                w411 = refnum<vi> refnum  # Boolean
                n206 = To More Specific Class(target class=w411, reference=w413) -> (specific class reference=w414:refnum<vi>)  [unwired: 1 in, 1 out]
                n207 = property class="Bool"(reference=w414, "BoolText.Text"=w412) -> ()  [unwired: 1 in, 2 out]
              }
              frame "FilterControl" {
                w417 = refnum<vi> refnum  # Boolean
                n208 = To More Specific Class(target class=w417, reference=w415) -> (specific class reference=w418:refnum<vi>)  [unwired: 1 in, 1 out]
                n209 = property class="Bool"(reference=w418, "BoolText.Text"=w416) -> ()  [unwired: 1 in, 2 out]
              }
              frame "AdjustedHeight" {
                n210 = property class="Ctl"(reference=w419, "Caption.Text"=w420) -> ()  [unwired: 1 in, 2 out]
              }
              frame "ReportSelection" {
                w422 = refnum<vi> refnum  # Ring
                n211 = To More Specific Class(target class=w422, reference=w424) -> (specific class reference=w423:refnum<vi>)  [unwired: 1 in, 1 out]
                n212 = property class="Ring"(reference=w423, "Caption.Text"=w425, "Strings []"=w421) -> ()  [unwired: 1 in, 2 out]
              }
              frame "GenerateReport" {
                w429 = refnum<vi> refnum  # Boolean
                n213 = To More Specific Class(target class=w429, reference=w427) -> (specific class reference=w428:refnum<vi>)  [unwired: 1 in, 1 out]
                n214 = property class="Bool"(reference=w428, "BoolText.Text"=w426) -> ()  [unwired: 1 in, 2 out]
              }
              frame "Remove Measurement Button" {
                w433 = refnum<vi> refnum  # Boolean
                n215 = To More Specific Class(target class=w433, reference=w431) -> (specific class reference=w432:refnum<vi>)  [unwired: 1 in, 1 out]
                n216 = property class="Bool"(reference=w432, "BoolText.Text"=w430) -> ()  [unwired: 1 in, 2 out]
              }
              frame "Data Listbox" {
                w436 = refnum<vi> refnum  # MulticolumnListbox
                n217 = To More Specific Class(target class=w436, reference=w435) -> (specific class reference=w437:refnum<vi>, error out=w438:errorcluster)  [unwired: 1 in]
                n218 = property class="MCListbox"(reference=w437, error in=w438, "ColHdrString"=w434) -> ()  [unwired: 2 out]
              }
              frame "ChangePassword" {
                w442 = refnum<vi> refnum  # Boolean
                n219 = To More Specific Class(target class=w442, reference=w439) -> (specific class reference=w441:refnum<vi>)  [unwired: 1 in, 1 out]
                n220 = property class="Bool"(reference=w441, "BoolText.Text"=w440) -> ()  [unwired: 1 in, 2 out]
              }
            }
          }
        }
        n221 = Transpose 2D Array(2D array=w264) -> (transposed array=→"Array":string[][])
        n222 = for {
          tunnel: w260 -> [w269] mode=indexing
          tunnel: w259 -> [w268] mode=indexing
          # "Tab captions"
          n223 = property class="Page"(reference=w269, "IndependentLabel"=TRUE ("Independent Label"), "TabCaption"=w268) -> ()  [unwired: 1 in, 2 out]
        }
      }
    }
  }
  n224 = Transpose 2D Array(2D array=w102) -> (transposed array=→"appended array":string[][])
